vi "DM delete bursts.vi"(9 "bursts to delete":string[](array[string]), 10 "group":string, 11 "module loopdata in":T1) -> (3 "module loopdata out":T1)   [LabVIEW 2019, in "DataManagment.lvlib"]
uses:
  DataManagment.lvlib
  module data.ctl
  SubVIs/mmWave data_class/mmWave data.lvclass
  DM signal group.ctl
  <userlib>/_OpenG.lib/array/array.llb/Delete Elements from 1D Array (String)__ogtk.vi
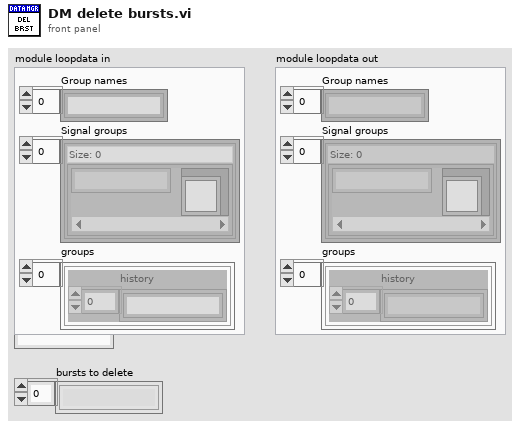
[diagram p1: front panel]
types:
  T1 = typedef "DataManagment.lvlib/module data.ctl" = cluster{"Group names":string[], "Signal groups":map{string, refnum<class "mmWave data.lvclass">}[], "groups":T2[]}
  T2 = typedef "DataManagment.lvlib/DM signal group.ctl" = cluster{"history":string[]}
  T3 = map{string, refnum<class "mmWave data.lvclass">}[]
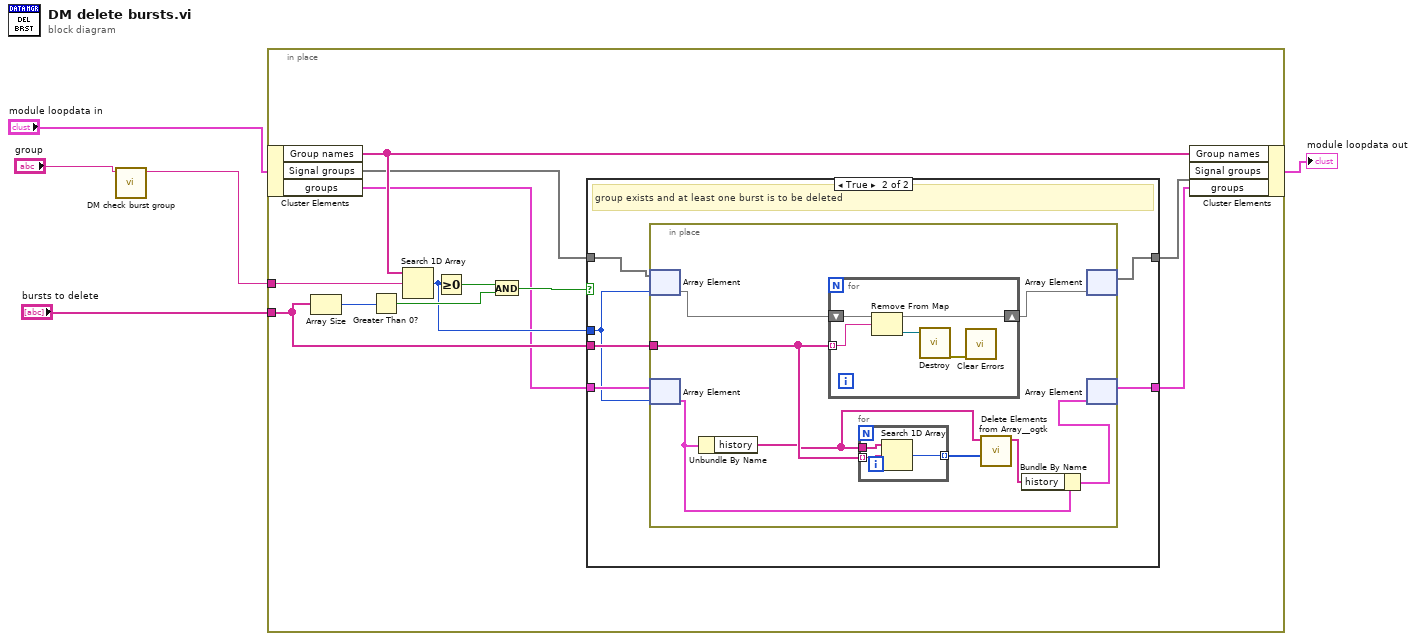
[diagram p0: block diagram]
diagram:
  n1 = call "DM check burst group.vi"("group"="group") -> ("String"=w3:string)  [unwired: 10 in]
  n2 = in-place {
    in-place-border: w3 -> [w17]
    in-place-border: "bursts to delete" -> [w9]
    n3 = in-place-cluster #1("module loopdata in") -> ("Group names"=w16:string[], "Signal groups"=w11:T3, "groups"=w7:T2[])
    n4 = Array Size(array=w9) -> (size(s)=w14:i32)
    n5 = Greater Than 0?(x=w14) -> (x > 0?=w13:bool)
    n6 = Search 1D Array(1D array=w16, element=w17) -> (index of element=w12:i32)  [unwired: 1 in]
    n7 = Greater Or Equal To 0?(x=w12) -> (x >= 0?=w15:bool)
    n8 = And(x=w15, y=w13) -> (x .and. y?=w10:bool)
    n9 = case shown="True" w10 {
      tunnel: w12 -> [_ w20]
      tunnel: w11 -> [w19 w24]
      tunnel: w9 -> [_ w25]
      tunnel: [w19 w23] -> w8
      tunnel: w7 -> [w18 w22]
      tunnel: [w18 w21] -> w6
      frame False {
      }
      frame True {
        # "group exists and at least one burst is to be deleted"
        n10 = in-place {
          in-place-border: w25 -> [w31]
          n11 = in-place-array #2(w24, w20) -> (w33:map{string, refnum<class "mmWave data.lvclass">})
          n12 = in-place-array #3(w22, w20) -> (w28:T2)
          n13 = Unbundle By Name(w28) -> ("history"=w30:string[])
          n14 = for {
            tunnel: w31 -> [w40] mode=indexing
            shift-right: [w37] -> w32
            shift-left: w33 -> [w41]
            n15 = Remove From Map(10:w40, 11:w41) -> (1:w39:refnum<class "mmWave data.lvclass">, 3:w37:map{string, refnum<class "mmWave data.lvclass">})  [unwired: 1 out]
            n16 = call-dynamic "Destroy.vi"("reference in"=w39) -> ("error out"=w38:errorcluster)  [unwired: 17 in, 1 out]
            n17 = call <vilib>:"Clear Errors.vi"("error in (no error)"=w38) -> ()  [unwired: 5 in, 2 out]
          }
          n18 = for {
            tunnel: w30 -> [w36]
            tunnel: w31 -> [w35] mode=indexing
            tunnel: [w34] -> w29 mode=indexing
            n19 = Search 1D Array(1D array=w36, element=w35) -> (index of element=w34:i32)  [unwired: 1 in]
          }
          n20 = call-poly <userlib>:"Delete Elements from Array__ogtk.vi"("indices"=w29, "array"=w30) -> ("array w/ subset deleted"=w27:string[])  [unwired: 8 in, 1 out]
          n21 = Bundle By Name(cluster=w28, "history"=w27) -> (w26:T2)
          n22 = in-place-array #2(w32) -> (w23:T3)  [unwired: 1 out]
          n23 = in-place-array #3(w26) -> (w21:T2[])  [unwired: 1 out]
        }
      }
    }
    n24 = in-place-cluster #1("Group names"=w16, "Signal groups"=w8, "groups"=w6) -> (→"module loopdata out":T1)
  }
